vi "Stop Acquisition.vi"(8 "error in":errorcluster, 11 "ImageHandler in":refnum<class "ImageHandler.lvclass">) -> (0 "error out":errorcluster, 3 "ImageHandler out":refnum<class "ImageHandler.lvclass">)   [LabVIEW 2022 SP3, in "ImageHandler.lvlib" / "ImageHandler.lvclass"]
uses:
  ImageHandler.lvclass
  ImageHandler.lvclass/ImageHandler.ctl
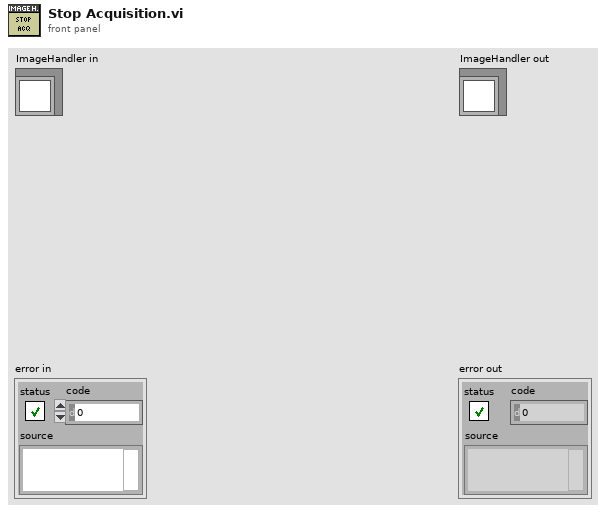
[diagram p1: front panel]
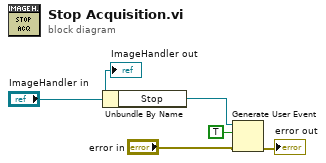
[diagram p0: block diagram]
diagram:
  n1 = Unbundle By Name("ImageHandler in") -> ("Stop"=w2:refnum<user-event>)
  n2 = Generate User Event(user event=w2, event data cluster=TRUE ("event data"), error in="error in") -> (error out=→"error out":errorcluster)  [unwired: 1 in, 1 out]
  "ImageHandler out" <- "ImageHandler in"
